vi "Get Device Information.vi"(8 "error in":errorcluster, 11 "VISA resource name in":refnum<visa-resource-name>) -> (0 "error out":errorcluster, 1 "Serial Number":string caption="Número de serie", 2 "Model Number":string caption="Número de modelo", 3 "VISA resource name out":refnum<visa-resource-name>, 4 "Firmware Revision":string, 5 "Manufacturer":string caption="Manufacturador")   [LabVIEW 2021, in "Keysight U1282A.lvlib"]
doc: "El comando de identificación (*IDN?) permite al instrumento U1281A/U1282A identificarse al proporcionar el número de modelo, el número de serie y la versión de firmware."
uses:
  Keysight U1282A.lvlib
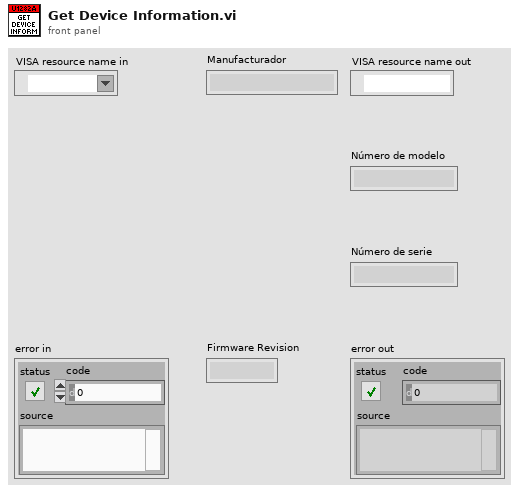
[diagram p1: front panel]
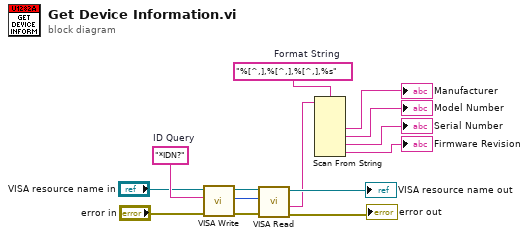
[diagram p0: block diagram]
diagram:
  w3 = "*IDN?"  # ID Query
  w14 = "%[^,],%[^,],%[^,],%s"  # Format String
  n1 = call "VISA Write.vi"("error in"="error in", "SCPI command"=w3, "VISA resource in"="VISA resource name in") -> ("error out"=w7:errorcluster, "Bytes at Port out"=w8:u32, "VISA resource out"=w9:refnum<visa-resource-name>)  [unwired: 6 in]
  n2 = call "VISA Read.vi"("error in"=w7, "Bytes at Port in"=w8, "VISA resource in"=w9) -> ("error out"=→"error out":errorcluster, "Reading"=w1:string, "VISA resource out"=→"VISA resource name out":refnum<visa-resource-name>)  [unwired: 5 in, 1 out]
  n3 = Scan From String(format string=w14, input string=w1) -> (output 1=→"Manufacturer":string, output 2=→"Model Number":string, output 3=→"Serial Number":string, output 4=→"Firmware Revision":string)  [unwired: 6 in, 3 out]
